vi "Set Arm State.vi"(8 "Error In":errorcluster) -> ()   [LabVIEW 2014]
uses:
  <vilib>/Platform/TimedLoop/XDataNode/timing_clust.ctl
  <vilib>/Platform/TimedLoop/XDataNode/nitl_modes.ctl
  <vilib>/Platform/TimedLoop/XDataNode/wakeup.ctl
  Web Services/DronePi Global Variables.vi
  <vilib>/platform/TimedLoop/XDataNode/XDataNode.xnode
  <vilib>/Platform/TimedLoop/XDataNode/XDNodeRunTimeDep.lvlib
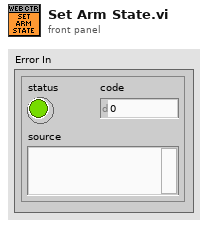
[diagram p1: front panel]
types:
  T1 = typedef "XDNodeRunTimeDep.lvlib/timing_clust.ctl" = cluster{"Expected End [f-1]":u64, "Actual End [f-1]":u64, "Finished Late? [f-1]":bool, "Expected End [i-1]":u64, "Actual End [i-1]":u64, "Finished Late? [i-1]":bool, "Expected Start [i]":u64, "Actual Start [i]":u64, "Expected Start [f]":u64, "Actual Start [f]":u64, "Source Name":string, "Structure Name":string, "Period":i64, "Deadline":i64, "Offset":i64, "Start":i64, "Priority":i32, "Timeout":i32, "Mode":T2, "Wakeup Reason":T3, "Error":errorcluster, "Source Type":string, "Secondary Source Type":string, "Global End Time":u64, "Global Start Time":u64, "Frame Duration":u64, "Iteration Duration":u64, "Assigned CPU":i32, "I/O Scan Engine Mode":u32}
  T2 = typedef "XDNodeRunTimeDep.lvlib/nitl_modes.ctl" = enum32{"No Change", "Process missed periods, maintain original phase", "Discard missed periods, maintain original phase", "Process missed periods, ignore original phase", "Discard missed periods, ignore original phase"}
  T3 = typedef "XDNodeRunTimeDep.lvlib/wakeup.ctl" = enum32{"Normal", "Aborted", "Asynchronous wakeup", "Timing source error", "Timed loop error", "Timeout"}
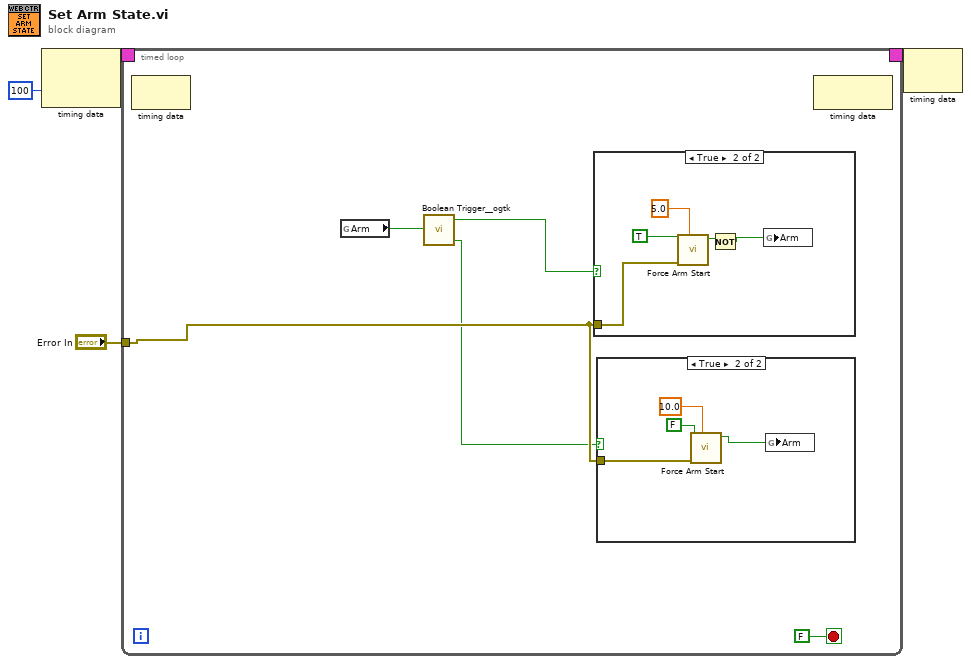
[diagram p0: block diagram]
diagram:
  n1 = node-c288(i64 100 ("Period")) -> (w4:T1)  [unwired: 1 in]
  n2 = timed-loop {
    timing: w4 -> [_]
    timing-out: [_] -> w3
    tunnel: "Error In" -> [w6]
    stop <- FALSE stop-if-true
    n3 = node-c288() -> ()  [unwired: 1 in, 1 out]
    n4 = global read "DronePi Global Variables.vi" "Arm"() -> (w8:bool)
    n5 = call <userlib>:"Boolean Trigger__ogtk.vi"("Boolean Input"=w8) -> ("Rising Edge"=w7:bool, "Falling Edge"=w5:bool)  [unwired: 1 in]
    n6 = case shown="True" w7 {
      tunnel: w6 -> [_ w16]
      frame False {
      }
      frame True {
        n7 = call "Force Arm Start.vi"("Timeout (s)"=5.0, "Error In"=w16, "ARM(T)/DISARM(F)"=TRUE) -> ("Time out"=w15:bool)  [unwired: 7 in, 1 out]
        n8 = Not(x=w15) -> (.not. x?=w14:bool)
        n9 = global write "DronePi Global Variables.vi" "Arm"(w14) -> ()
      }
    }
    n10 = case shown="True" w5 {
      tunnel: w6 -> [_ w11]
      frame False {
      }
      frame True {
        n11 = call "Force Arm Start.vi"("Timeout (s)"=10.0, "Error In"=w11, "ARM(T)/DISARM(F)"=FALSE) -> ("Time out"=w10:bool)  [unwired: 7 in, 1 out]
        n12 = global write "DronePi Global Variables.vi" "Arm"(w10) -> ()
      }
    }
    n13 = node-c288() -> ()  [unwired: 1 in, 1 out]
  }
  n14 = node-c288(w3) -> ()  [unwired: 1 out]
